vi "Assignment 08.05.2020.vi"() -> ()   [LabVIEW 2019]
panel:
  out "Result":bool
  in  "B":bool
  in  "A":bool
  out "min(x,y)":dbl
  out "max(x,y)":dbl
  in  "Int 4":dbl
  in  "Int 3":dbl
  out "Result":bool
  in  "Int 2":dbl
  in  "Int1":dbl
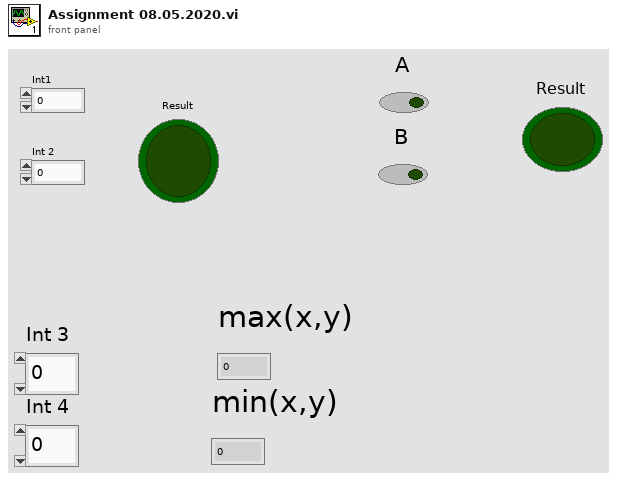
[diagram p1: front panel]
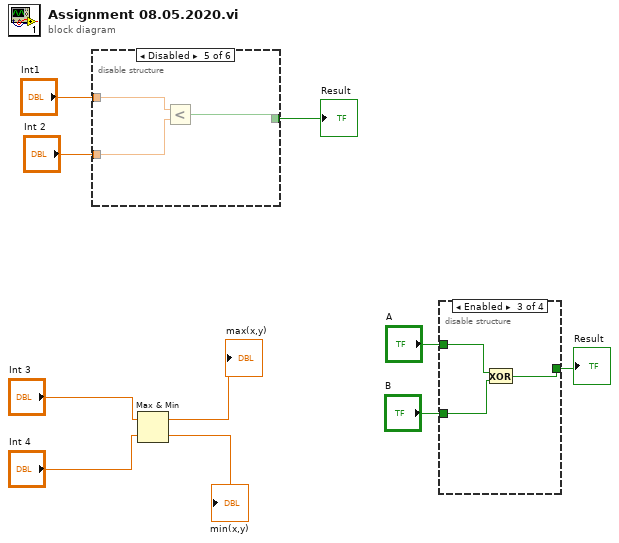
[diagram p0: block diagram]
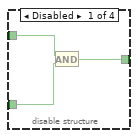
[diagram p2: hidden frame]
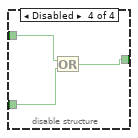
[diagram p4: hidden frame]
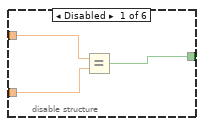
[diagram p5: hidden frame]
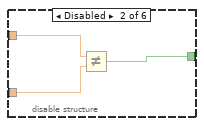
[diagram p6: hidden frame]
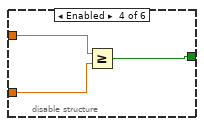
[diagram p8: hidden frame]
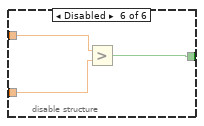
[diagram p9: hidden frame]
diagram:
  n1 = disable-structure shown="Disabled" {
    disable-tunnel: "Int1" -> [w13 w16 _ w19 w22 w25]
    disable-tunnel: "Int 2" -> [w12 w15 _ w18 w21 w24]
    disable-tunnel: [w11 w14 _ w17 w20 w23] -> w9
    frame Disabled {
      n2 = Equal?(x=w13, y=w12) -> (x = y?=w11:bool)
    }
    frame Disabled {
      n3 = Not Equal?(x=w16, y=w15) -> (x != y?=w14:bool)
    }
    frame Disabled {
    }
    frame Enabled {
      n4 = Greater Or Equal?(x=w19, y=w18) -> (x >= y?=w17:bool)
    }
    frame Disabled {
      n5 = Less?(x=w22, y=w21) -> (x < y?=w20:bool)
    }
    frame Disabled {
      n6 = Greater?(x=w25, y=w24) -> (0:w23:bool)
    }
  }
  "Result" <- w9
  n7 = Max & Min(x="Int 3", y="Int 4") -> (max(x,y)=→"max(x,y)":dbl, min(x,y)=→"min(x,y)":dbl)
  n8 = disable-structure shown="Enabled" {
    disable-tunnel: "A" -> [w28 _ w31 w34]
    disable-tunnel: "B" -> [w27 _ w30 w33]
    disable-tunnel: [w26 _ w29 w32] -> w1
    frame Disabled {
      n9 = And(x=w28, y=w27) -> (x .and. y?=w26:bool)
    }
    frame Disabled {
    }
    frame Enabled {
      n10 = Exclusive Or(1:w30, 2:w31) -> (0:w29:bool)
    }
    frame Disabled {
      n11 = Or(x=w34, y=w33) -> (x .or. y?=w32:bool)
    }
  }
  "Result" <- w1
